vi "流程写入.vi"(10 "简易流程路径":path, 11 "添加的路径":path caption="测试流程路径") -> ()   [LabVIEW 2016, in "斯坦道氟化物.lvlib"]
uses:
  <vilib>/Utility/miscctls.llb/LVPointTypeDef.ctl
panel:
  in  "选项卡控件":enum32{"测试流程", "简易流程"}(tab)
  in  "一键写入":bool
  in  "量程下拉列表":enum16{"低量程", "高量程"}(ring)
  in  "测量模式":T1(ring)
  in  "简易流程":u16(ring)
  in  "一键写入 2":bool=TRUE
  in  "关闭":bool
  out "字符串":string
  in  "写入":bool
  in  "参数下拉列表":u16(ring)
  # "请选择要写入的流程"
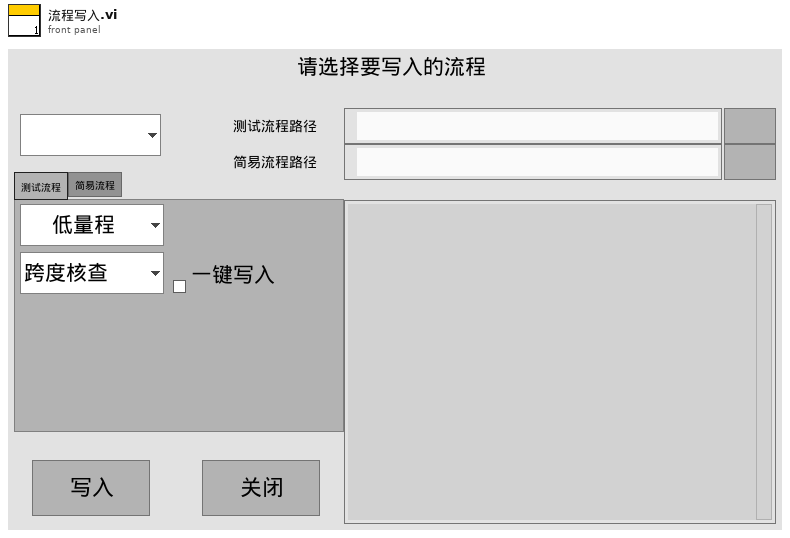
[diagram p1: front panel]
types:
  T1 = enum16{"跨度核查", "水样测量", "零点核查", "标样核查", "加标回收", "快捷测试", "空白校准", "标样校准"}
  T2 = typedef "LVPointTypeDef.ctl" = cluster{"Horizontal":i16, "Vertical":i16}
  T3 = typedef "LVStringsAndValuesArrayTypeDef_U16.ctl" = cluster{"String":string, "Value":u16}[]
  T4 = typedef "操作日志字段定义.ctl" = cluster{"时间":timestamp, "参数":string, "日志信息":string, "流程参数":string}
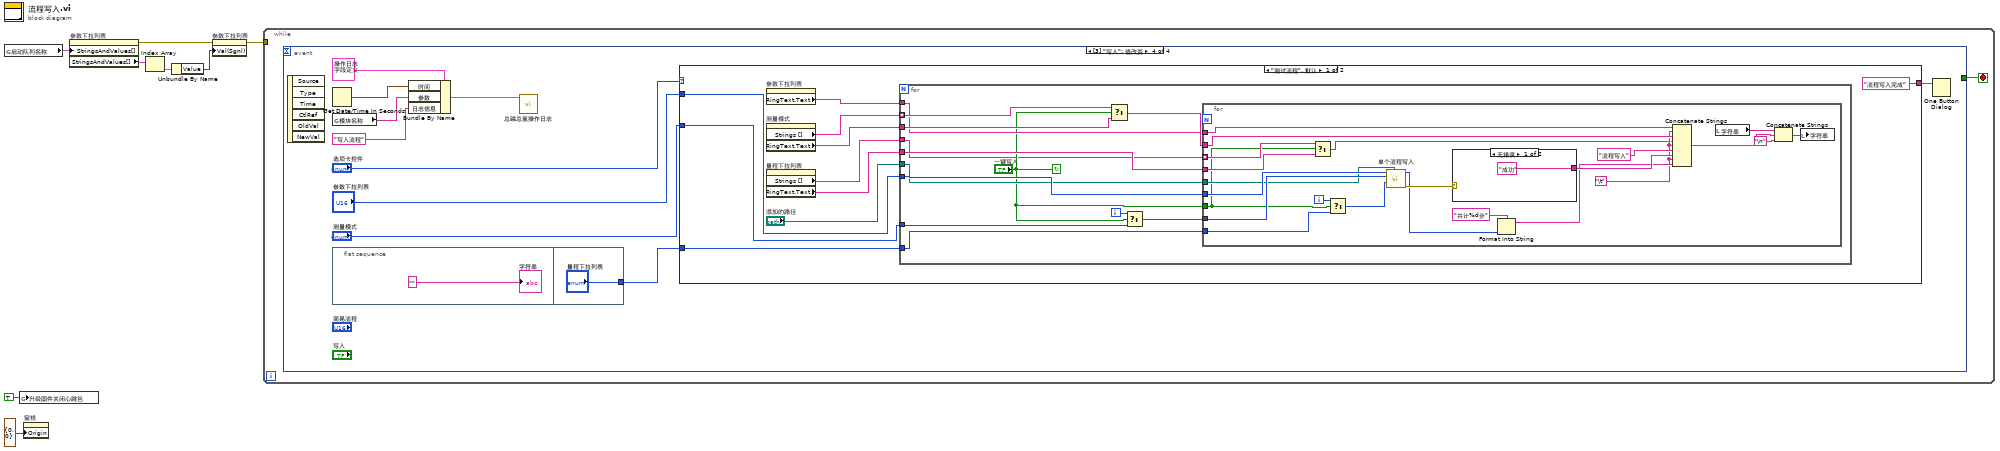
[diagram p0: block diagram]
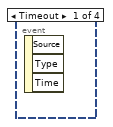
[diagram p2: hidden frame]
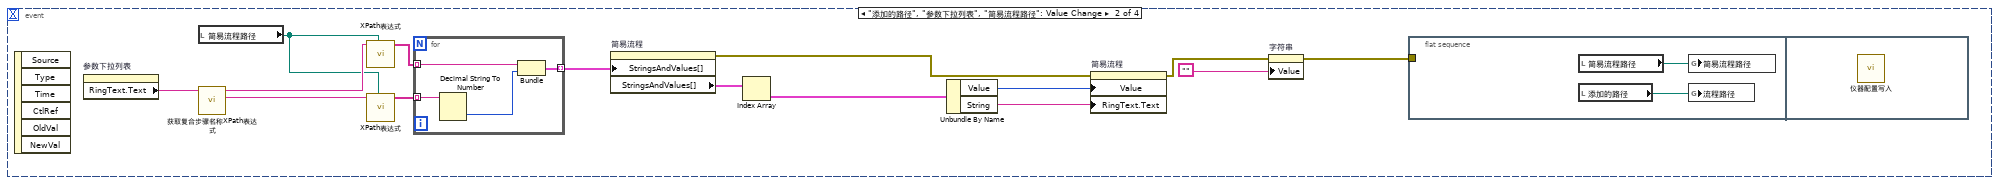
[diagram p3: hidden frame]
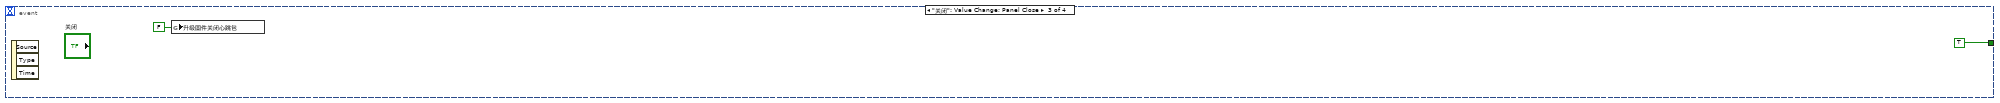
[diagram p4: hidden frame]
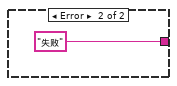
[diagram p5: hidden frame]
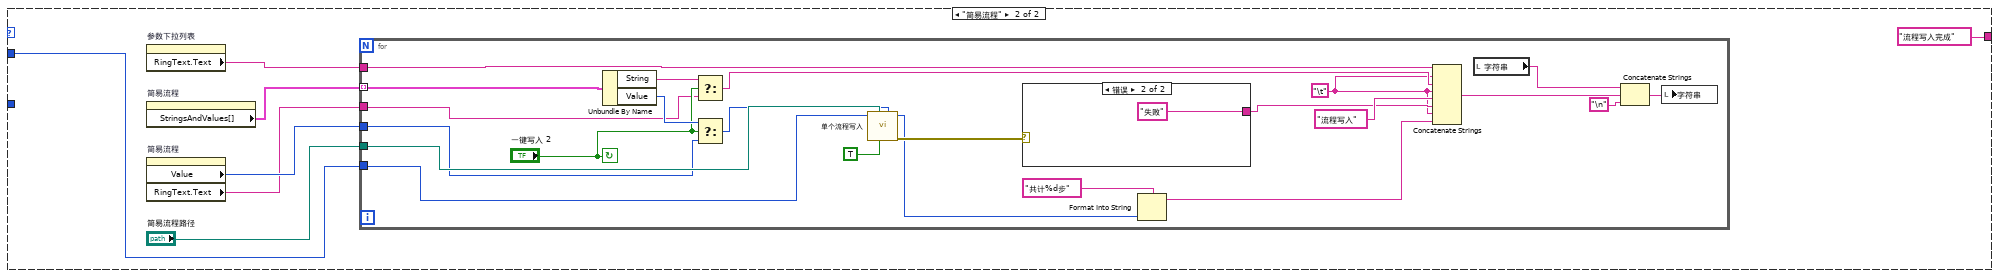
[diagram p6: hidden frame]
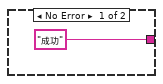
[diagram p7: hidden frame]
diagram:
  n1 = global read "model config var.vi" "启动队列名称"() -> (w7:cluster{"String":string, "Value":u16}[])
  n2 = global write "VAR总磷总氮全局变量.vi" "升级固件关闭心跳包"(TRUE ("升级固件关闭心跳包")) -> ()
  n3 = property on="窗格" class="Pane"("Origin"=T2 {"Horizontal"=0, "Vertical"=0} ("原点")) -> ()  [unwired: 2 in, 2 out]
  n4 = property on="参数下拉列表" class="Ring (严格)"("StringsAndValues[]"=w7) -> (error out=w6:errorcluster, "StringsAndValues[]"=w5:T3)  [unwired: 2 in, 1 out]
  n5 = Index Array(array=w5) -> (element=w4:cluster{"String":string, "Value":u16})  [unwired: 1 in]
  n6 = Unbundle By Name(w4) -> ("Value"=w3:u16)
  n7 = property on="参数下拉列表" class="Ring (严格)"(error in=w6, "Val(Sgnl)"=w3) -> (error out=w2:errorcluster)  [unwired: 1 in, 1 out]
  n8 = while {
    tunnel: w2 -> [_]
    stop <- w9 stop-if-true
    n9 = event shown="[3] \"写入\": 值改变" {
      selector: _ -> [_ _ _ _]
      dyn-events: _ -> [_ _ _ _]
      timeout: _ -> [_ _ _ _]
      tunnel: [_ _ TRUE _] -> w9
      event Timeout {
        n10 = event-data() -> ()  [unwired: 1 in, 3 out]
      }
      event "添加的路径", "参数下拉列表", "简易流程路径": Value Change {
        n11 = event-data() -> ()  [unwired: 1 in, 6 out]
        n12 = property on="参数下拉列表" class="Ring (严格)"() -> ("RingText.Text"=w23:string)  [unwired: 2 in, 2 out]
        n13 = local read "简易流程路径"() -> (w17:path)
        n14 = call "获取复合步骤名称XPath表达式.vi"("查询参数"=w23) -> ("FlowId"=w22:string, "name"=w24:string)  [unwired: 9 in]
        n15 = call "XPath表达式.vi"("添加的路径"=w17, "XPath expression"=w24) -> ("数组"=w21:string[])  [unwired: 9 in]
        n16 = call "XPath表达式.vi"("添加的路径"=w17, "XPath expression"=w22) -> ("数组"=w20:string[])  [unwired: 9 in]
        n17 = for {
          tunnel: w21 -> [w30] mode=indexing
          tunnel: w20 -> [w29] mode=indexing
          tunnel: [w27] -> w19 mode=indexing
          n18 = Decimal String To Number(string=w29) -> (number=w28:i32)  [unwired: 2 in, 1 out]
          n19 = Bundle("node text"=w30, w28) -> (w27:cluster{"node text":string, i32})  [unwired: 1 in]
        }
        n20 = property on="简易流程" class="Ring (严格)"("StringsAndValues[]"=w19) -> (error out=w16:errorcluster, "StringsAndValues[]"=w14:T3)  [unwired: 2 in, 1 out]
        n21 = Index Array(array=w14) -> (element=w13:cluster{"String":string, "Value":u16})  [unwired: 1 in]
        n22 = Unbundle By Name(w13) -> ("Value"=w12:u16, "String"=w10:string)
        n23 = property on="简易流程" class="Ring (严格)"(error in=w16, "Value"=w12, "RingText.Text"=w10) -> (error out=w15:errorcluster)  [unwired: 1 in, 1 out]
        n24 = property on="字符串" class="Str"(error in=w15, "Value"="") -> (error out=w11:errorcluster)  [unwired: 1 in, 1 out]
        n25 = flat-sequence {
          tunnel: w11 -> [_]
          frame #0 {
            n26 = local read "简易流程路径"() -> (w26:path)
            n27 = local read "添加的路径"() -> (w25:path)
            n28 = global write "总磷总氮断电保存全局变量.vi" "简易流程路径"(w26) -> ()
            n29 = global write "总磷总氮断电保存全局变量.vi" "流程路径"(w25) -> ()
          }
          frame #1 {
            n30 = call "仪器配置写入.vi"() -> ()  [unwired: 11 in, 1 out]
          }
        }
      }
      event "关闭": Value Change; Panel Close {
        n31 = event-data() -> ()  [unwired: 1 in, 3 out]
        n32 = global write "VAR总磷总氮全局变量.vi" "升级固件关闭心跳包"(FALSE ("升级固件关闭心跳包")) -> ()
      }
      event "写入": Value Change {
        n33 = event-data() -> ()  [unwired: 1 in, 6 out]
        n34 = Get Date/Time In Seconds() -> (seconds since 1Jan1904=w35:timestamp)
        n35 = global read "VAR总磷总氮全局变量.vi" "模块名称"() -> (w33:string)
        n36 = flat-sequence {
          tunnel: ["量程下拉列表"] -> w41
          frame #0 {
            "字符串" <- ""
          }
          frame #1 {
          }
        }
        n37 = Bundle By Name(cluster=T4 {"时间"=timestamp(0 s since 1904-01-01), "参数"="", "日志信息"="", "流程参数"=""} ("data in"), "时间"=w35, "参数"=w33, "日志信息"="写入流程") -> (w36:T4)
        n38 = call "总磷总氮操作日志.vi"("data in"=w36) -> ()  [unwired: 10 in, 1 out]
        n39 = case shown="\"测试流程\", 默认" "选项卡控件" {
          tunnel: "参数下拉列表" -> [w50 w97]
          tunnel: w41 -> [w51 _]
          tunnel: ["流程写入完成" ("消息") "流程写入完成" ("消息")] -> w39
          tunnel: "测量模式" -> [w48 _]
          frame "测试流程", Default {
            n40 = property on="参数下拉列表" class="Ring (严格)"() -> ("RingText.Text"=w45:string)  [unwired: 2 in, 2 out]
            n41 = property on="测量模式" class="Enum (严格)"() -> ("Strings []"=w49:string[], "RingText.Text"=w46:string)  [unwired: 2 in, 2 out]
            n42 = property on="量程下拉列表" class="Enum (严格)"() -> ("Strings []"=w43:string[], "RingText.Text"=w47:string)  [unwired: 2 in, 2 out]
            n43 = for {
              tunnel: w51 -> [w65]
              tunnel: w50 -> [w63]
              tunnel: w49 -> [w59] mode=indexing
              tunnel: w48 -> [w62]
              tunnel: w47 -> [w60]
              tunnel: w46 -> [w58]
              tunnel: "添加的路径" -> [w56]
              tunnel: w45 -> [w55]
              tunnel: w43 -> [w53]
              i -> [w64]
              stop <- "一键写入" continue-if-true
              n44 = Select(t=w59, s="一键写入", f=w58) -> (s? t:f=w57:string)
              n45 = Select(t=w64, s="一键写入", f=w62) -> (s? t:f=w61:i32)
              n46 = for {
                tunnel: w65 -> [w81]
                tunnel: w63 -> [w80]
                tunnel: w61 -> [w79]
                tunnel: w60 -> [w68]
                tunnel: w57 -> [w78]
                tunnel: w56 -> [w77]
                tunnel: w55 -> [w76]
                tunnel: "一键写入" -> [w66]
                tunnel: w53 -> [w69] mode=indexing
                i -> [w70]
                w72 = "\t"
                n47 = Select(t=w69, s=w66, f=w68) -> (s? t:f=w67:string)
                n48 = Select(t=w70, s=w66, f=w81) -> (s? t:f=w71:i32)
                n49 = call "单个流程写入.vi"("添加的路径"=w77, "量程"=w71, "测量模式"=w79, "测量参数"=w80) -> ("error out"=w88:errorcluster, "步数"=w75:i32)  [unwired: 5 in, 1 out]
                n50 = case shown="无错误" w88 {
                  tunnel: ["成功" "失败"] -> w85
                  frame No Error {
                  }
                  frame Error {
                  }
                }
                n51 = Format Into String(format string="共计%d步" ("格式字符串"), w75) -> (resulting string=w73:string)  [unwired: 2 in, 1 out]
                n52 = Concatenate Strings(w76, w72, w78, w67, w72, "流程写入", w85, w72, w73) -> (w84:string)
                n53 = local read "字符串"() -> (w87:string)
                n54 = Concatenate Strings(w87, w84, "\n") -> (w82:string)
                n55 = local write "字符串"(w82) -> ()
              }
            }
          }
          frame "简易流程" {
            n56 = property on="参数下拉列表" class="Ring (严格)"() -> ("RingText.Text"=w91:string)  [unwired: 2 in, 2 out]
            n57 = property on="简易流程" class="Ring (严格)"() -> ("StringsAndValues[]"=w96:T3)  [unwired: 2 in, 2 out]
            n58 = property on="简易流程" class="Ring (严格)"() -> ("Value"=w94:u16, "RingText.Text"=w93:string)  [unwired: 2 in, 2 out]
            n59 = for {
              tunnel: w96 -> [w110] mode=indexing
              tunnel: "简易流程路径" -> [w113]
              tunnel: w97 -> [w112]
              tunnel: w94 -> [w107]
              tunnel: w93 -> [w104]
              tunnel: w91 -> [w98]
              stop <- "一键写入 2" continue-if-true
              w99 = "\t"
              n60 = Unbundle By Name(w110) -> ("String"=w105:string, "Value"=w109:u16)
              n61 = Select(t=w105, s="一键写入 2", f=w104) -> (s? t:f=w103:string)
              n62 = Select(t=w109, s="一键写入 2", f=w107) -> (s? t:f=w108:u16)
              n63 = call "单个流程写入.vi"("简易流程Id"=w108, "是否是简易流程"=TRUE, "添加的路径"=w113, "测量参数"=w112) -> ("error out"=w120:errorcluster, "步数"=w102:i32)  [unwired: 5 in, 1 out]
              n64 = case shown="错误" w120 {
                tunnel: ["成功" "失败"] -> w117
                frame No Error {
                }
                frame Error {
                }
              }
              n65 = Format Into String(format string="共计%d步" ("格式字符串"), w102) -> (resulting string=w100:string)  [unwired: 2 in, 1 out]
              n66 = Concatenate Strings(w98, w99, w103, w99, "流程写入", w117, w99, w100) -> (w116:string)
              n67 = local read "字符串"() -> (w119:string)
              n68 = Concatenate Strings(w119, w116, "\n") -> (w114:string)
              n69 = local write "字符串"(w114) -> ()
            }
          }
        }
        n70 = One Button Dialog(message=w39) -> ()  [unwired: 1 in, 1 out]
      }
    }
  }
